vi "Do This.vi"(8 "error in (no error)":errorcluster, 10 "Status Events":refnum<class "Status Events.lvclass">, 11 "Run VI in":refnum<class "Run VI.lvclass">) -> (0 "error out":errorcluster, 3 "Run VI out":refnum<class "Run VI.lvclass">)   [LabVIEW 2014, in "Run VI.lvclass"]
uses:
  Run VI.lvclass
  Classes/Status Events/Status Events.lvclass
  Run VI.lvclass/Run VI.ctl
  <vilib>/Utility/error.llb/DialogType.ctl
  Classes/Job/Job.lvclass/Job.ctl
  Classes/Job/Job.lvclass
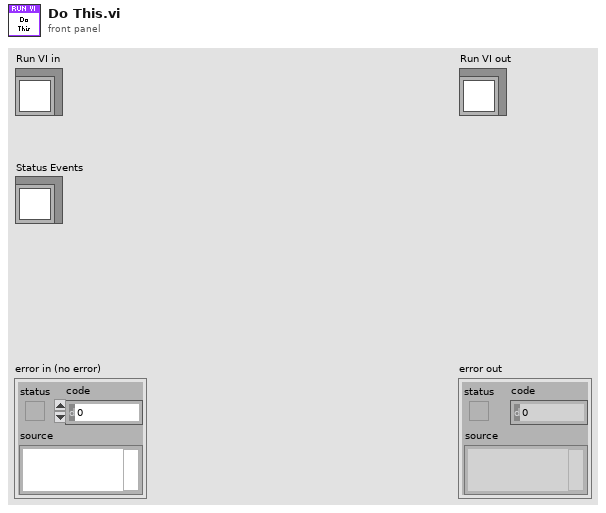
[diagram p1: front panel]
types:
  T1 = typedef "DialogType.ctl" = u16
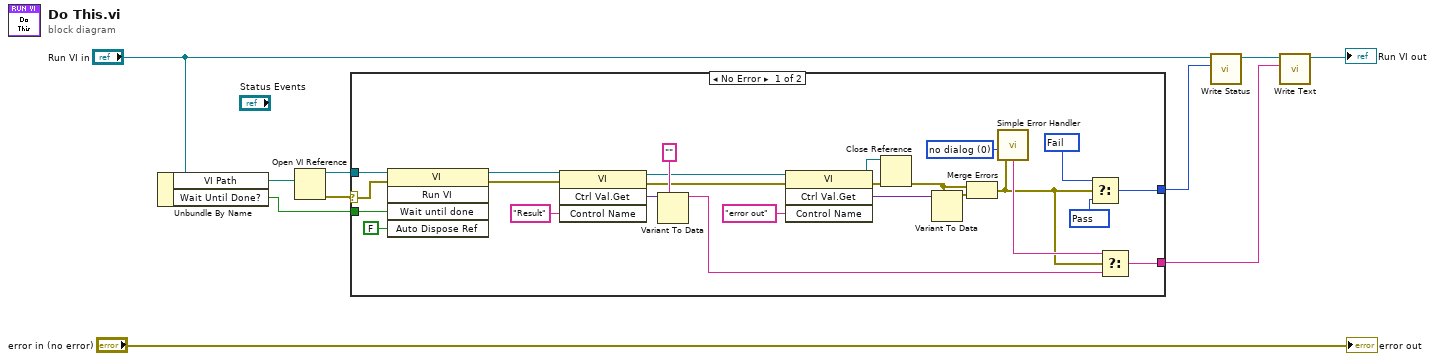
[diagram p0: block diagram]
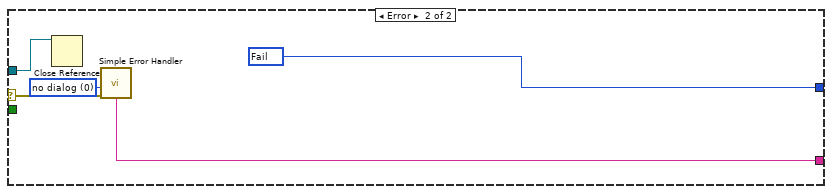
[diagram p2: hidden frame]
diagram:
  n1 = Unbundle By Name("Run VI in") -> ("VI Path"=w7:path, "Wait Until Done?"=w4:bool)
  n2 = Open VI Reference(vi path=w7) -> (vi reference=w6:refnum<vi>, error out=w5:errorcluster)  [unwired: 5 in]
  n3 = case shown="No Error" w5 {
    selector: w5 -> [w17 w40]
    tunnel: w6 -> [w35 w36]
    tunnel: w4 -> [w34 _]
    tunnel: [w21 w38] -> w2
    tunnel: [w24 w37] -> w3
    frame No Error {
      w19 = u16 200 items=["Service Error"=504, "Abort"=503, "Fail"=500, "Pass"=200] ("Status")
      w26 = T1 0 items=["no dialog", "OK message", "continue or stop message", "OK message + warnings", "continue/stop + warnings"] ("type of dialog (OK msg:1)")
      w25 = u16 500 items=["Service Error"=504, "Abort"=503, "Fail"=500, "Pass"=200] ("Status")
      n4 = invoke class="VI" method="Run VI"(reference=w35, error in=w17, "Wait until done"=w34, "Auto Dispose Ref"=FALSE ("Auto Dispose Reference")) -> (reference out=w33:refnum<vi>, error out=w16:errorcluster)  [unwired: 1 in, 3 out]
      n5 = invoke class="VI" method="Ctrl Val.Get"(reference=w33, error in=w16, "Control Name"="Result") -> (reference out=w28:refnum<vi>, error out=w15:errorcluster, "Get Control Value Variant"=w31:variant)  [unwired: 1 in, 1 out]
      n6 = Variant To Data(type="", Variant=w31) -> (data=w20:string)  [unwired: 1 in, 1 out]
      n7 = invoke class="VI" method="Ctrl Val.Get"(reference=w28, error in=w15, "Control Name"="error out") -> (reference out=w11:refnum<vi>, error out=w13:errorcluster, "Get Control Value Variant"=w27:variant)  [unwired: 1 in, 1 out]
      n8 = Close Reference(reference=w11, error in (no error)=w13) -> (error out=w12:errorcluster)
      n9 = Variant To Data(type=w12, Variant=w27) -> (data=w23:errorcluster)  [unwired: 1 in, 1 out]
      n10 = Merge Errors(w12, w23) -> (w14:errorcluster)
      n11 = call <vilib>:"Simple Error Handler.vi"("type of dialog (OK msg:1)"=w26, "error in (no error)"=w14) -> ("message"=w22:string)  [unwired: 3 in, 4 out]
      n12 = Select(t=w25, s=w14, f=w19) -> (s? t:f=w24:u16)
      n13 = Select(t=w22, s=w14, f=w20) -> (s? t:f=w21:string)
    }
    frame Error {
      w37 = u16 500 items=["Service Error"=504, "Abort"=503, "Fail"=500, "Pass"=200] ("Status")
      w39 = T1 0 items=["no dialog", "OK message", "continue or stop message", "OK message + warnings", "continue/stop + warnings"] ("type of dialog (OK msg:1)")
      n14 = Close Reference(reference=w36) -> ()  [unwired: 1 in, 1 out]
      n15 = call <vilib>:"Simple Error Handler.vi"("type of dialog (OK msg:1)"=w39, "error in (no error)"=w40) -> ("message"=w38:string)  [unwired: 3 in, 4 out]
    }
  }
  n16 = call "Write Status.vi"("Status"=w3, "Job in"="Run VI in") -> ("Job out"=w10:refnum<class "Run VI.lvclass">)  [unwired: 8 in, 1 out]
  n17 = call "Write Text.vi"("Text"=w2, "Job in"=w10) -> ("Job out"=→"Run VI out":refnum<class "Run VI.lvclass">)  [unwired: 8 in, 1 out]
  "error out" <- "error in (no error)"
